vi "System.vi"() -> ()   [LabVIEW 2020]
uses:
  Global_Variable/Global.vi
panel:
  in  "excursion":T1
  # "偏移设置"
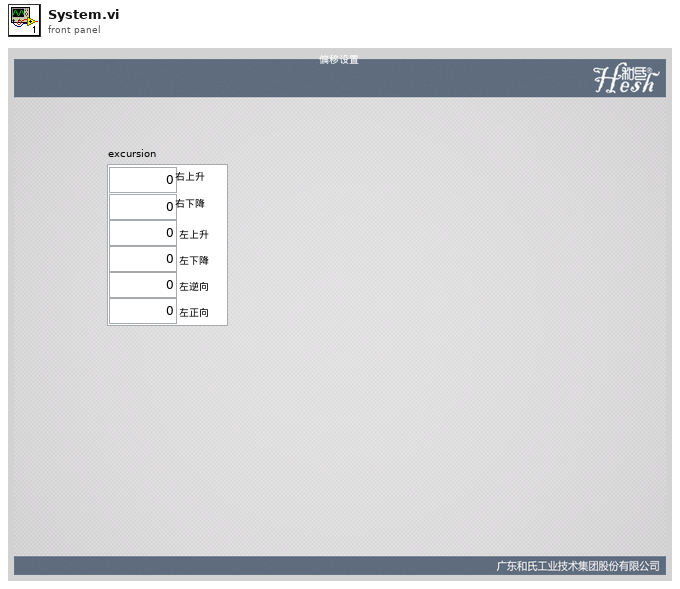
[diagram p1: front panel]
types:
  T1 = cluster{"右上升":dbl, "右下降":dbl, "左上升":dbl, "左下降":dbl, "左逆向":dbl, "左正向":dbl}
  T2 = typedef "System_conf.ctl" = cluster{"右上升":dbl, "右下降":dbl, "左上升":dbl, "左下降":dbl, "左逆向":dbl, "左正向":dbl}
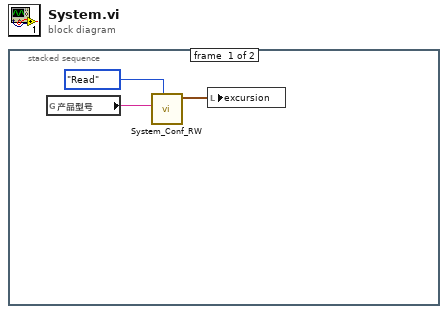
[diagram p0: block diagram]
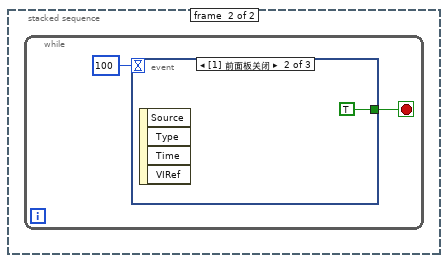
[diagram p2: hidden frame]
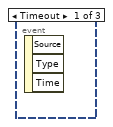
[diagram p3: hidden frame]
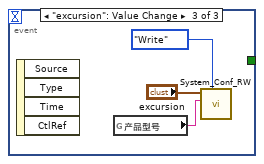
[diagram p4: hidden frame]
diagram:
  n1 = stacked-sequence {
    frame #0 {
      n2 = global read "Global.vi" "产品型号"() -> (w1:string)
      n3 = call "System_Conf_RW.vi"("Mode"=enum16{"Read", "Write"}."Read", "Section"=w1) -> ("excursion_out"=w3:T2)  [unwired: 8 in, 1 out]
      n4 = local write "excursion"(w3) -> ()
    }
    frame #1 {
      n5 = while {
        stop <- w5 stop-if-true
        n6 = event shown="[1] 前面板关闭" {
          selector: _ -> [_ _ _]
          dyn-events: _ -> [_ _ _]
          timeout: 100 -> [_ _ _]
          tunnel: [_ TRUE _] -> w5
          event Timeout {
            n7 = event-data() -> ()  [unwired: 1 in, 3 out]
          }
          event Panel Close {
            n8 = event-data() -> ()  [unwired: 1 in, 4 out]
          }
          event "excursion": Value Change {
            n9 = event-data() -> ()  [unwired: 1 in, 4 out]
            n10 = global read "Global.vi" "产品型号"() -> (w7:string)
            n11 = call "System_Conf_RW.vi"("Mode"=enum16{"Read", "Write"}."Write", "Section"=w7, "excursion"="excursion") -> ()  [unwired: 7 in, 2 out]
          }
        }
      }
    }
  }
